vi "BRig_dataLC_Wrong_Prob_l1.vi"() -> (2 "output_Wrong_Prob":i32)   [LabVIEW 2014]
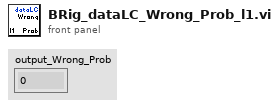
[diagram p1: front panel]
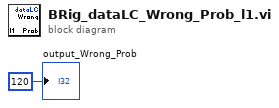
[diagram p0: block diagram]
diagram:
  "output_Wrong_Prob" <- 120 ("output_iBlock")
